vi "Teleop Cmd Changed.vi"(8 "Epsilon":dbl, 10 "New Teleop Values":T1, 11 "Prev Teleop Values":T1) -> (3 "Boolean":bool)   [LabVIEW 2013]
uses:
  TeleopCmd.ctl
  robot/Lightning/CmdFlag.ctl
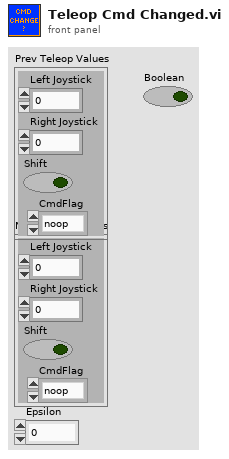
[diagram p1: front panel]
types:
  T1 = typedef "TeleopCmd.ctl" = cluster{"Left Joystick":dbl, "Right Joystick":dbl, "Shift":bool, "CmdFlag":T2}
  T2 = typedef "CmdFlag.ctl" = enum16{"noop", "suspend", "resume"}
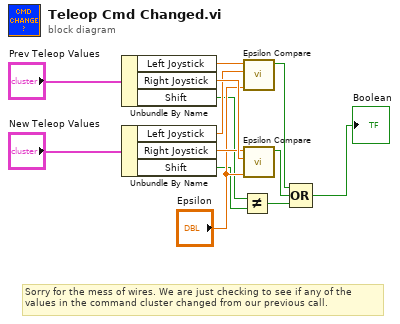
[diagram p0: block diagram]
diagram:
  # "Sorry for the mess of wires. We are just checking to see if any of the \nvalues in the command cluster changed from our previous call."
  n1 = Unbundle By Name("Prev Teleop Values") -> ("Left Joystick"=w10:dbl, "Right Joystick"=w13:dbl, "Shift"=w6:bool)
  n2 = Unbundle By Name("New Teleop Values") -> ("Left Joystick"=w9:dbl, "Right Joystick"=w12:dbl, "Shift"=w5:bool)
  n3 = Not Equal?(x=w6, y=w5) -> (x != y?=w2:bool)
  n4 = call "Epsilon Compare.vi"("Epsilon"="Epsilon", "Value2"=w9, "Value1"=w10) -> ("Boolean"=w4:bool)  [unwired: 8 in]
  n5 = call "Epsilon Compare.vi"("Epsilon"="Epsilon", "Value2"=w13, "Value1"=w12) -> ("Boolean"=w3:bool)  [unwired: 8 in]
  n6 = Compound Arithmetic op=OR(w4, w3, w2) -> (→"Boolean":bool)
